vi "ISX3_ClearBuffer.vi"(3 "Handle":u32) -> (0 "Bytes Read from the buffer":u32, 1 "Handle":u32)   [LabVIEW 2012, in "Sciospec ISX3 Impedance Analyzer.lvlib"]
uses:
  Sciospec ISX3 Impedance Analyzer.lvlib
panel:
  out "Buffer":u8[](array[numeric])
  # "This VI reads and dicards all available bytes currently waiting in the USB buffer."
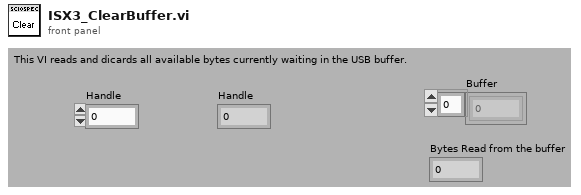
[diagram p1: front panel]
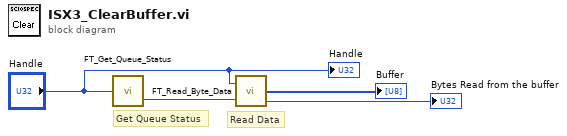
[diagram p0: block diagram]
diagram:
  # "Read Data"
  # "Get Queue Status"
  n1 = call "FT_Get_Queue_Status.vi"("Handle"="Handle") -> ("Bytes Waiting"=w4:u32)  [unwired: 1 out]
  n2 = call "FT_Read_Byte_Data.vi"("Handle"="Handle", "Bytes To Read"=w4) -> ("Read Data"=→"Buffer":u8[], "Bytes Read"=→"Bytes Read from the buffer":u32)  [unwired: 1 out]
  "Handle" <- "Handle"
